vi "Draw_Grid.vi"(7 "Grid Line Color":u32(colorbox)=16760386, 8 "error in (no error)":errorcluster, 10 "Grid Lines":u32=2, 11 "Image In":T1) -> (0 "error out":errorcluster, 3 "Image Out":T1)   [LabVIEW 2020]
doc: "This example program overlays a grid on an image, displays it in an image display and writes a JPEG file with the grid overlay information. Follow the steps below to run the vi:\n\n1. Select an image file\n2. Select the spacing in pixels between grid lines\n3. Select the grid line color\n4. Run the VI"
uses:
  <vilib>/vision/Image Controls.llb/IMAQ Image.ctl
panel:
  out "Y Resolution":i32
  out "X Resolution":i32
  out "For Itr 2":i32
  out "For Itr1":i32
  out "Image":T1(plugin-control)
  out "Grid Line Spacing":u32=100
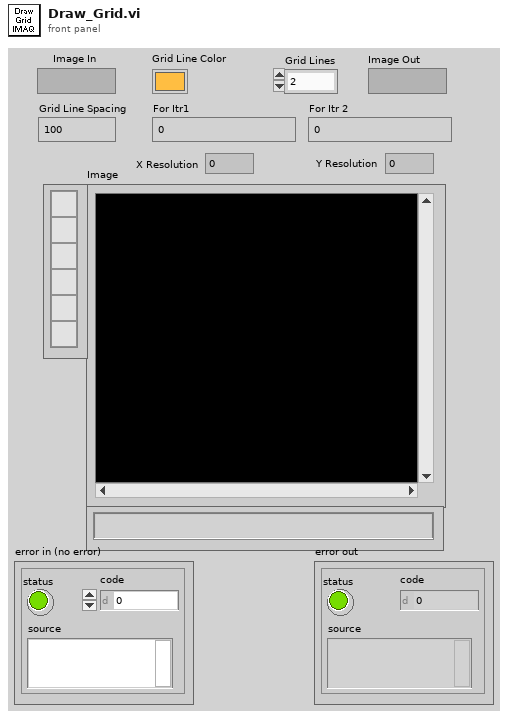
[diagram p1: front panel]
types:
  T1 = typedef "IMAQ Image.ctl" = refnum<image>
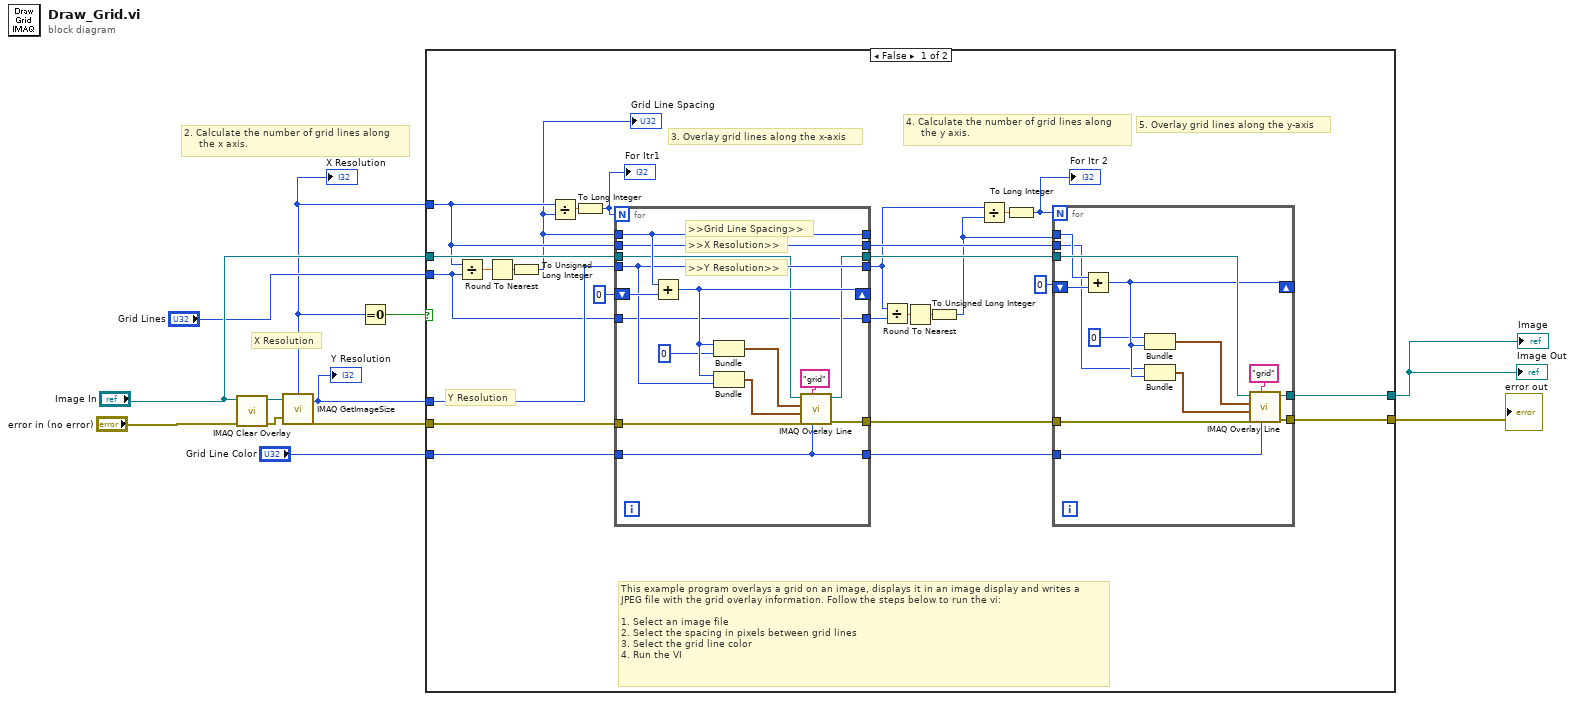
[diagram p0: block diagram]
diagram:
  # "X Resolution"
  # "2. Calculate the number of grid lines along\n     the x axis."
  n1 = call "IMAQ Clear Overlay"("error in (no error)"="error in (no error)", "Image"="Image In") -> ("error out"=w4:errorcluster, "Image Out"=w6:T1)  [unwired: 8 in]
  n2 = call "IMAQ GetImageSize"("Image"=w6, "error in (no error)"=w4) -> ("Y Resolution"=w10:i32, "X Resolution"=w2:i32, "error out"=w12:errorcluster)  [unwired: 2 in]
  "X Resolution" <- w2
  "Y Resolution" <- w10
  n3 = Equal To 0?(x=w2) -> (x = 0?=w1:bool)
  n4 = case shown="False" w1 {
    tunnel: w12 -> [w38 w67]
    tunnel: "Image In" -> [w36 w68]
    tunnel: w10 -> [w31 _]
    tunnel: "Grid Line Color" -> [w26 _]
    tunnel: [w24 w68] -> w8
    tunnel: [w23 w67] -> w7
    tunnel: w2 -> [w20 _]
    tunnel: "Grid Lines" -> [w16 _]
    frame False {
      # "This example program overlays a grid on an image, displays it in an image display and writes a \nJPEG file with the grid overlay information. Follow the steps below to run the vi:\n\n1. Select an image file\n2. Select the spacing in pixels between grid lines\n3. Select the grid line color\n4. Run the VI"
      # "Y Resolution"
      # "5. Overlay grid lines along the y-axis"
      # "4. Calculate the number of grid lines along\n     the y axis."
      # "3. Overlay grid lines along the x-axis"
      n5 = Divide(x=w20, y=w16) -> (x/y=w22:dbl)
      n6 = Round To Nearest(number=w22) -> (nearest integer value=w21:dbl)
      n7 = To Unsigned Long Integer(number=w21) -> (unsigned 32bit integer=w19:u32)
      "Grid Line Spacing" <- w19
      n8 = Divide(x=w20, y=w19) -> (x/y=w34:dbl)
      n9 = To Long Integer(number=w34) -> (32bit integer=w33:i32)
      "For Itr1" <- w33
      n10 = for {
        N: w33 -> [_]
        tunnel: w38 -> [w66]
        tunnel: [w65] -> w37
        tunnel: w36 -> [w54]
        tunnel: [w55] -> w35
        tunnel: w19 -> [w64]
        tunnel: [w64] -> _
        tunnel: [w60] -> w14
        tunnel: w31 -> [w60]
        shift-right: [w62] -> _
        shift-left: 0 -> [w63]
        tunnel: [w57] -> w28
        tunnel: w20 -> [w57]
        tunnel: w26 -> [w56]
        tunnel: [w56] -> w25
        tunnel: w16 -> [w53]
        tunnel: [w53] -> w15
        # ">>Y Resolution>>"
        # ">>X Resolution>>"
        # ">>Grid Line Spacing>>"
        n11 = Add(x=w64, y=w63) -> (x+y=w62:u32)
        n12 = Bundle(w62, 0) -> (w59:cluster{u32, i32})  [unwired: 1 in]
        n13 = Bundle(w62, "Y Resolution"=w60) -> (w58:cluster{u32, "Y Resolution":i32})  [unwired: 1 in]
        n14 = call "IMAQ Overlay Line"("Color"=w56, "Group"="grid", "error in (no error)"=w66, "End Point"=w58, "Start Point"=w59, "Image"=w54) -> ("error out"=w65:errorcluster, "Image Out"=w55:T1)  [unwired: 4 in]
      }
      n15 = Divide(x=w14, y=w15) -> (x/y=w17:dbl)
      n16 = Round To Nearest(number=w17) -> (nearest integer value=w18:dbl)
      n17 = To Unsigned Long Integer(number=w18) -> (unsigned 32bit integer=w13:u32)
      n18 = Divide(x=w14, y=w13) -> (x/y=w32:dbl)
      n19 = To Long Integer(number=w32) -> (32bit integer=w27:i32)
      "For Itr 2" <- w27
      n20 = for {
        N: w27 -> [_]
        tunnel: w37 -> [w51]
        tunnel: [w50] -> w23
        tunnel: w35 -> [w49]
        shift-right: [w46] -> _
        shift-left: 0 -> [w48]
        tunnel: w13 -> [w47]
        tunnel: w28 -> [w44]
        tunnel: [w41] -> w24
        tunnel: w25 -> [w40]
        n21 = Add(x=w47, y=w48) -> (x+y=w46:u32)
        n22 = Bundle(0, w46) -> (w43:cluster{i32, u32})  [unwired: 1 in]
        n23 = Bundle("X Resolution"=w44, w46) -> (w42:cluster{"X Resolution":i32, u32})  [unwired: 1 in]
        n24 = call "IMAQ Overlay Line"("Color"=w40, "Group"="grid", "error in (no error)"=w51, "End Point"=w42, "Start Point"=w43, "Image"=w49) -> ("error out"=w50:errorcluster, "Image Out"=w41:T1)  [unwired: 4 in]
      }
    }
    frame True {
    }
  }
  "Image" <- w8
  "error out" <- w7
  "Image Out" <- w8
